vi "List Files Under Project Folder.vi"() -> ()   [LabVIEW 2020]
uses:
  File/File.lvclass/File.lvclass/File.ctl
  LabVIEW File/LabVIEW File.lvclass
  LabVIEW File/LabVIEW File.lvclass/LabVIEW File.ctl
  LabVIEW File/Read Version String.vi
  File/File.lvclass/Read Path.vi
  File/File.lvclass/Read is LabVIEW File Type.vi
  <userlib>/_OpenG.lib/file/file.llb/Compare Two Paths - Scalar__ogtk.vi
  File/File.lvclass/File.lvclass
  <vilib>/Utility/lvfile.llb/NI_FileType.lvlib
panel:
  out "concatenated string 2":string
  out "concatenated string":string
  out "error out":errorcluster
  in  "Files":i32(listbox)
  in  "Save for LabVIEW Version":string
  in  "Project Folder":path
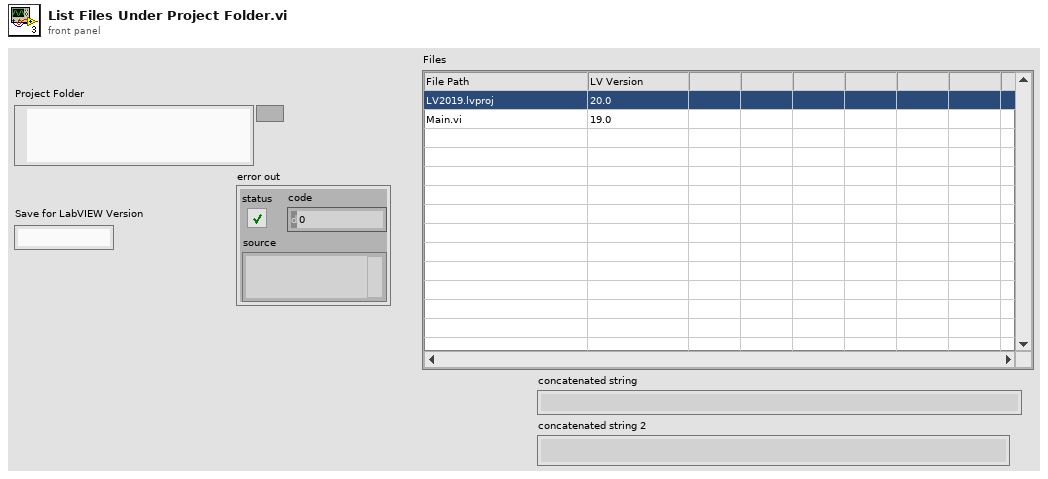
[diagram p1: front panel]
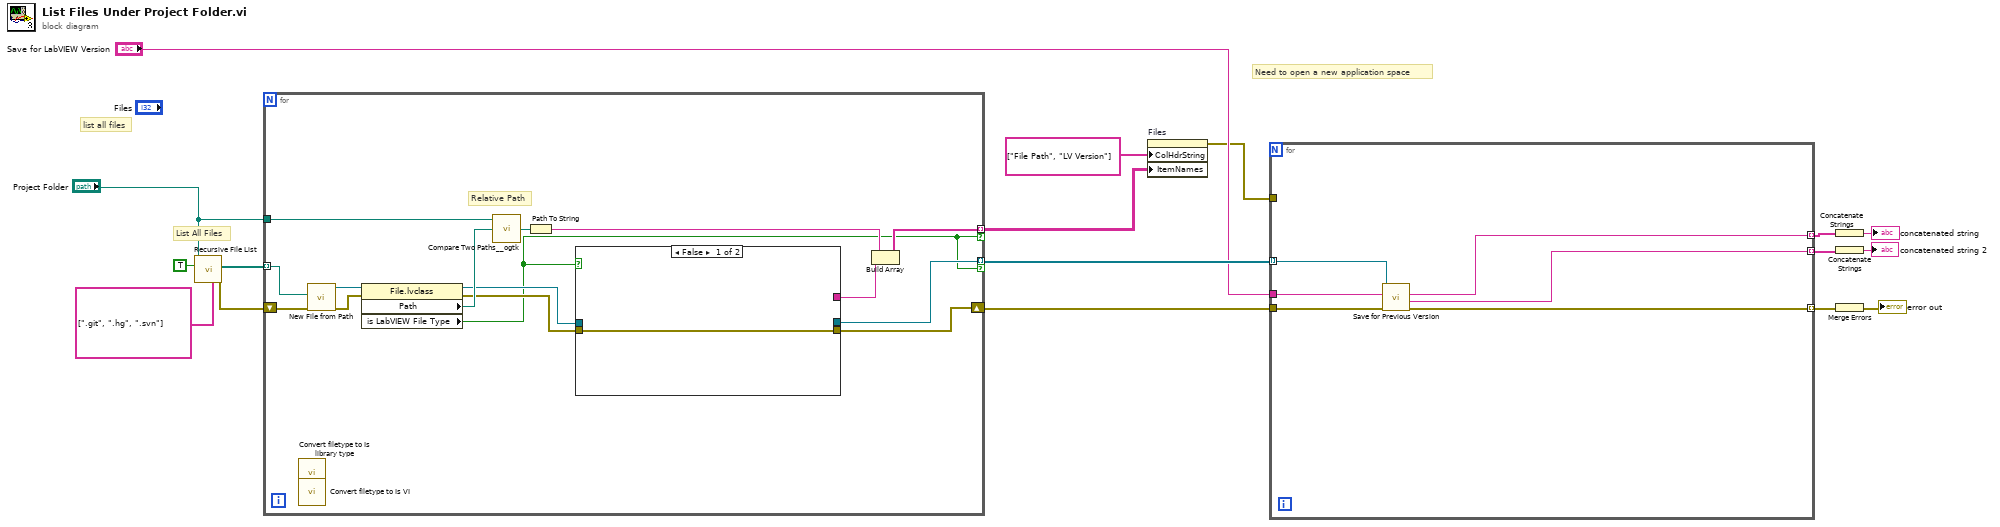
[diagram p0: block diagram]
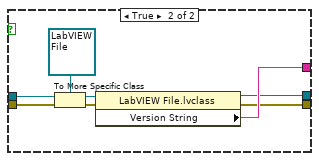
[diagram p2: hidden frame]
diagram:
  # "List All Files"
  # "Need to open a new application space"
  # "list all files"
  n1 = call <vilib>:"Recursive File List.vi"("Folders to Exclude"=string[] [".git", ".hg", ".svn"], "Treat LLBs as Folders?"=TRUE, "Folder Path"="Project Folder") -> ("error out"=w13:errorcluster, "All Files in Dir"=w15:path[])  [unwired: 4 in, 3 out]
  n2 = for {
    tunnel: w15 -> [w30] mode=indexing
    tunnel: "Project Folder" -> [w32]
    tunnel: [w22] -> w12 mode=indexing if=w18
    shift-right: [w21] -> w9
    shift-left: w13 -> [w26]
    tunnel: [w19] -> w10 mode=indexing if=w18
    # "Relative Path"
    n3 = call <vilib>:"Convert filetype to Is library type.vi"() -> ()  [unwired: 5 in, 1 out]
    n4 = call <vilib>:"Convert filetype to Is VI.vi"() -> ()  [unwired: 5 in, 1 out]
    n5 = call "New File from Path.vi"("error in (no error)"=w26, "Path"=w30) -> ("error out"=w27:errorcluster, "File out"=w29:refnum<class "File.lvclass">)  [unwired: 8 in]
    n6 = property class="File.lvclass"(reference=w29, error in=w27) -> (reference out=w25:refnum<class "File.lvclass">, error out=w20:errorcluster, "Path"=w28:path, "is LabVIEW File Type"=w18:bool)
    n7 = call-poly <userlib>:"Compare Two Paths__ogtk.vi"("path2"=w28, "path1"=w32) -> ("relative path from 1 to 2"=w31:path)  [unwired: 1 in, 2 out]
    n8 = Path To String(path=w31) -> (string=w23:string)
    n9 = case shown="False" w18 {
      tunnel: w25 -> [_ w40]
      tunnel: [_ w38] -> w24
      tunnel: [w33 w37] -> w21
      tunnel: w20 -> [w33 w35]
      tunnel: [_ w34] -> w19
      frame False {
      }
      frame True {
        n10 = To More Specific Class(target class=refnum<class "LabVIEW File.lvclass"> refnum ("Save for Previous Version.lvlib:LabVIEW File.lvclass"), reference=w40, error in=w35) -> (specific class reference=w39:refnum<class "LabVIEW File.lvclass">, error out=w36:errorcluster)
        n11 = property class="LabVIEW File.lvclass"(reference=w39, error in=w36) -> (reference out=w34:refnum<class "LabVIEW File.lvclass">, error out=w37:errorcluster, "Version String"=w38:string)
      }
    }
    n12 = Build Array(w23, w24) -> (w22:string[])
  }
  n13 = property on="Files" class="MCListbox (strict)"("ColHdrString"=string[] ["File Path", "LV Version"] ("Row Header Strings[]"), "ItemNames"=w12) -> (error out=w1:errorcluster)  [unwired: 2 in, 1 out]
  n14 = for {
    tunnel: w10 -> [w47] mode=indexing
    tunnel: w9 -> [w46]
    tunnel: [w45] -> w8 mode=indexing
    tunnel: [w44] -> w4 mode=indexing
    tunnel: [w43] -> w5 mode=indexing
    tunnel: "Save for LabVIEW Version" -> [w42]
    tunnel: w1 -> [_]
    n15 = call-dynamic "Save for Previous Version.vi"("error in (no error)"=w46, "LabVIEW Version"=w42, "LabVIEW File in"=w47) -> ("error out"=w45:errorcluster, "Errors"=w43:string, "Warnings"=w44:string)  [unwired: 5 in, 1 out]
  }
  n16 = Concatenate Strings(w4) -> (→"concatenated string":string)
  n17 = Concatenate Strings(w5) -> (→"concatenated string 2":string)
  n18 = Merge Errors(w8) -> (→"error out":errorcluster)
